vi "setImageBinning.vi"(8 "error in (no error)":errorcluster, 10 "Image Binning":T1={"Vertical Binning"=1.0, "Horizontal Binning"=1.0, "SubArea Height"=1024.0, "SubAreaWidth"=1024.0, "Offset"=0.0, "Mode"=FALSE, "Number of Tracks"=0.0, "Track Positions"=[], "subArea Coordinate"=[1.0, 1.0]}, 11 "CameraSettingsManager.lvclass in":refnum<class "CameraSettingsManager.lvclass">) -> (0 "error out":errorcluster, 3 "CameraSettingsManager.lvclass out":refnum<class "CameraSettingsManager.lvclass">)   [LabVIEW 2011, in "Tools.lvlib" / "Settings.lvlib" / "CameraSettingsManager.lvclass"]
uses:
  CameraSettingsManager.lvclass
  CameraSettingsManager.lvclass/CameraSettingsManager.ctl
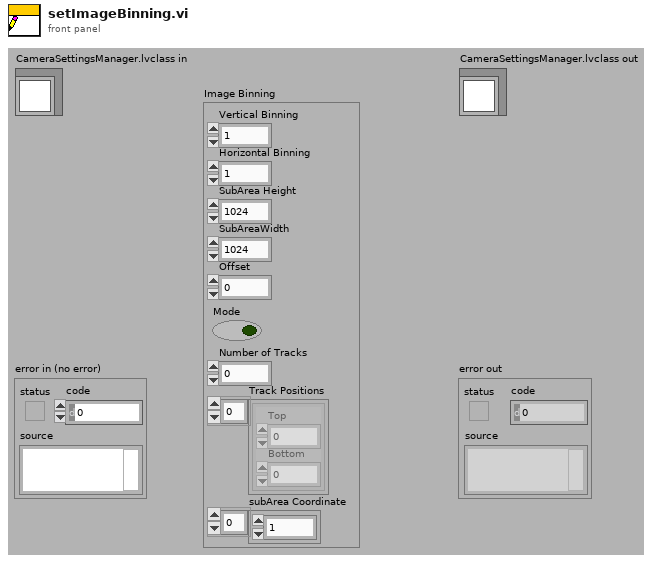
[diagram p1: front panel]
types:
  T1 = cluster{"Vertical Binning":dbl, "Horizontal Binning":dbl, "SubArea Height":dbl, "SubAreaWidth":dbl, "Offset":dbl, "Mode":bool, "Number of Tracks":dbl, "Track Positions":cluster{"Top":dbl, "Bottom ":dbl}[], "subArea Coordinate":dbl[]}
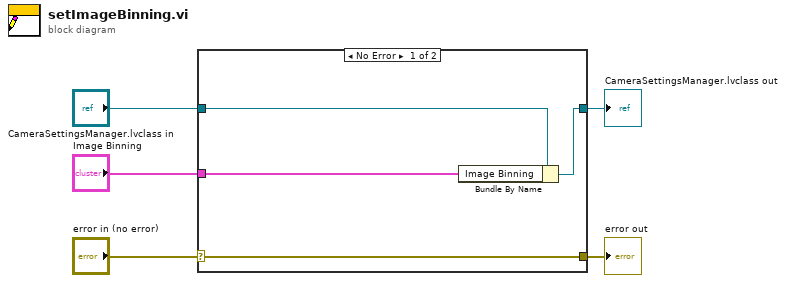
[diagram p0: block diagram]
diagram:
  n1 = case shown="No Error" "error in (no error)" {
    selector: "error in (no error)" -> [w9 w10]
    tunnel: [w9 w10] -> w4
    tunnel: [w7 w11] -> w2
    tunnel: "CameraSettingsManager.lvclass in" -> [w8 w11]
    tunnel: "Image Binning" -> [w6 _]
    frame No Error {
      n2 = Bundle By Name(cluster=w8, "Image Binning"=w6) -> (w7:refnum<class "CameraSettingsManager.lvclass">)
    }
    frame Error {
    }
  }
  "error out" <- w4
  "CameraSettingsManager.lvclass out" <- w2
